vi "Save niVNA Sweep Data to csv.vi"(4 "Meas Type":string="QuickView_", 5 "Selected Exp Settings":T13={"P2_Sweep_Stop_V"=36.0, "P2_Sweep_Step_V"=1.0, "Experiment Name"="", "Resistance Threshold"=1.0, "P1_Fixed_Voltage"=36.0, "P2_Sweep_Start_V"=36.0}, 6 "Additional Data":T14, 7 "Filepath":path, 8 "Parametric Calculated Values":T5={"Voltage Calculated Values"={"P1_VPD_C"=0.0, "P2_VPD_C"=0.0, "P1_VPD_Rel_C"=0.0, "P2_VPD_Rel_C"=0.0}, "Resistance Calculated Values"={"Rc_free"=0.0, "Rc_first"=0.0, "Rc_vmax"=0.0, "Rc_last"=0.0, "Rc_end"=0.0, "VPD_R"=0.0, "VPD_Rel_R"=0.0}, "Capacitance Calculated Values"={"P1_CPD_free"=0.0, "P2_CPD_free"=0.0, "P1_CPD_vmax"=0.0, "P2_CPD_vmax"=0.0, "P1_CPD_first"=0.0, "P2_CPD_first"=0.0, "P1_CPD_last"=0.0, "P2_CPD_last"=0.0, "P1_CPD_end"=0.0, "P2_CPD_end"=0.0, "P1_CPD_max"=0.0, "P2_CPD_max "=0.0, "CPD_Free"=0.0, "CPD_First"=0.0, "CPD_max"=0.0, "CPD_Last"=0.0, "CPD_End"=0.0, "CPD_vmax"=0.0}, "Cap Calc Arrays"={"CPD_sum"=[], "P2_CPD@V"=[], "P1_CPD@V"=[], "Specific Voltages"=[32.0, 36.0]}, "Resistance Array Calc"={"RC@V"=[]}, "TN4 Calc"={"P1_TN4_ACT"=0.0, "P2_TN4_ACT "=0.0, "VPD_R_2"=0.0, "DVR"=0.0}, "Corrected_Capacitance Calculated Values"={"P1_CPD_free"=0.0, "P2_CPD_free"=0.0, "P1_CPD_vmax"=0.0, "P2_CPD_vmax"=0.0, "P1_CPD_first"=0.0, "P2_CPD_first"=0.0, "P1_CPD_last"=0.0, "P2_CPD_last"=0.0, "P1_CPD_end"=0.0, "P2_CPD_end"=0.0, "P1_CPD_max"=0.0, "P2_CPD_max "=0.0, "CPD_Free"=0.0, "CPD_First"=0.0, "CPD_max"=0.0, "CPD_Last"=0.0, "CPD_End"=0.0, "CPD_vmax"=0.0}}, 9 "ks5080A_Meaurements":T4, 10 "Date Cluster":T3, 11 "Test Information":T2={"Exp Name"="Cold Switching", "Lot"="0233A", "Wafer"="15", "Die Type"="L22", "Die X "="6", "Die Y"="8", "Exp"="1", "Die X_Y"="8"}) -> ()   [LabVIEW 2013]
uses:
  Controls/Date Control.ctl
  Controls/Individual User Inputs.ctl
  Controls/Test Information.ctl
  Controls/Parametric Calculated Values.ctl
  Controls/Voltage Calculated Values.ctl
  Controls/Resistance Individual Calculated Values.ctl
  Controls/Capacitance Individual Calculated Values.ctl
  Controls/Capacitance Array Calculated Values.ctl
  Controls/Resistance Array Calculated Values.ctl
  Controls/TN4 Calc.ctl
  Controls/Corrected_Capacitance Individual Calculated Values.ctl
  Controls/Additional Data.ctl
  Controls/ks5080A_Measurements.ctl
  <vilib>/Utility/file.llb/Write To Spreadsheet File (string).vi
panel:
  in  "Tab Control":T1(tab)
  # "Test Settings"
  # "Make the Stop and Step Negative \nfor negative sweep"
  # "Calculation Settings"
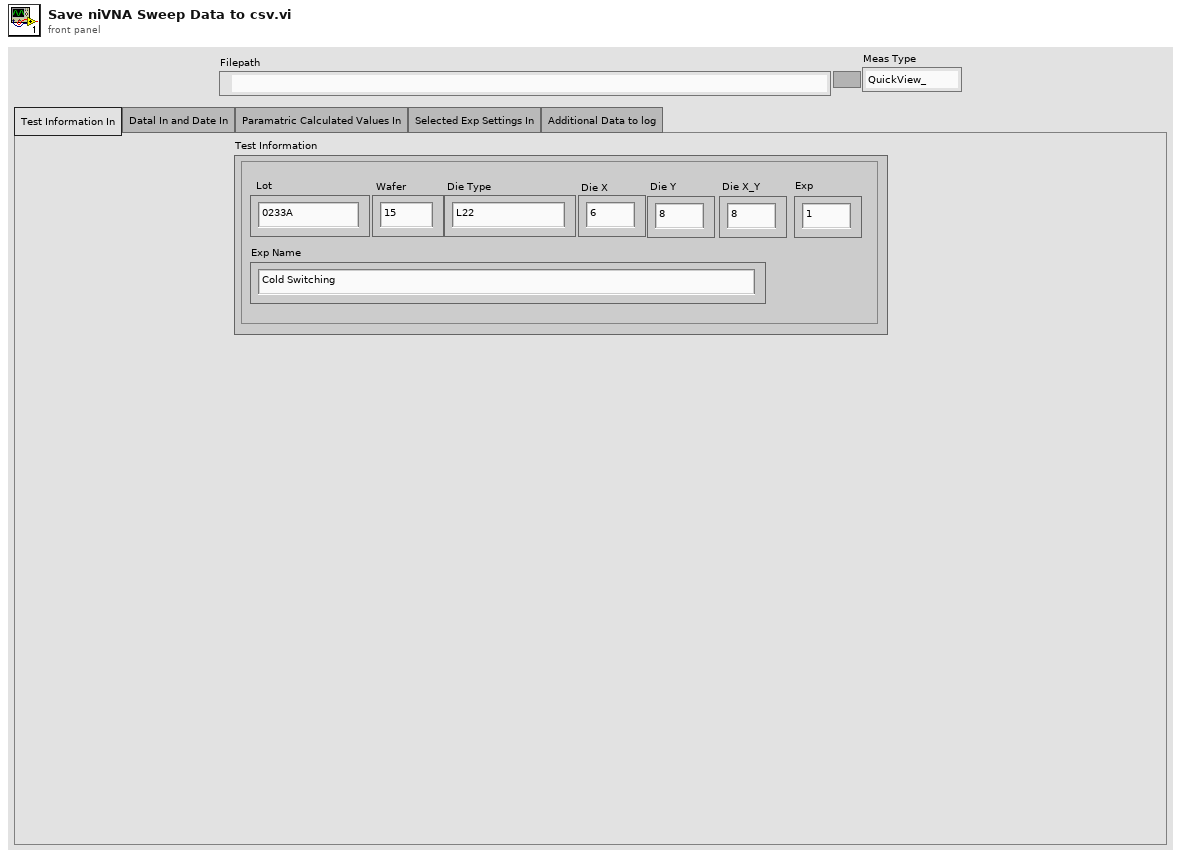
[diagram p1: front panel]
types:
  T1 = enum32{"Test Information In", "Datal In and Date In", "Paramatric Calculated Values In", "Selected Exp Settings In", "Additional Data to log"}
  T2 = typedef "Test Information.ctl" = cluster{"Exp Name":string, "Lot":string, "Wafer":string, "Die Type":string, "Die X ":string, "Die Y":string, "Exp":string, "Die X_Y":string}
  T3 = typedef "Date Control.ctl" = cluster{"Date":string, "Start Time":string, "Stop Time":string}
  T4 = typedef "ks5080A_Measurements.ctl" = cluster{"Bias_Sweep_Setting":dbl[], "Bias_voltage measurements":dbl[], "Bias_current measurements":dbl[], "P1_Capacitance":dbl[], "P2_Capacitance":dbl[], "DMM_Measurement_V":dbl[], "Contact_Source Current measurements":dbl[], "Contact_Sink Current measurements":dbl[], "Calculated_Resistance":dbl[], "P3_Capacitance":dbl[], "Port 1_S_parm":string[], "Port 2_S_parm":string[], "Port 3_S_parm":string[]}
  T5 = typedef "Parametric Calculated Values.ctl" = cluster{"Voltage Calculated Values":T6, "Resistance Calculated Values":T7, "Capacitance Calculated Values":T8, "Cap Calc Arrays":T9, "Resistance Array Calc":T10, "TN4 Calc":T11, "Corrected_Capacitance Calculated Values":T12}
  T6 = typedef "Voltage Calculated Values.ctl" = cluster{"P1_VPD_C":dbl, "P2_VPD_C":dbl, "P1_VPD_Rel_C":dbl, "P2_VPD_Rel_C":dbl}
  T7 = typedef "Resistance Individual Calculated Values.ctl" = cluster{"Rc_free":dbl, "Rc_first":dbl, "Rc_vmax":dbl, "Rc_last":dbl, "Rc_end":dbl, "VPD_R":dbl, "VPD_Rel_R":dbl}
  T8 = typedef "Capacitance Individual Calculated Values.ctl" = cluster{"P1_CPD_free":dbl, "P2_CPD_free":dbl, "P1_CPD_vmax":dbl, "P2_CPD_vmax":dbl, "P1_CPD_first":dbl, "P2_CPD_first":dbl, "P1_CPD_last":dbl, "P2_CPD_last":dbl, "P1_CPD_end":dbl, "P2_CPD_end":dbl, "P1_CPD_max":dbl, "P2_CPD_max ":dbl, "CPD_Free":dbl, "CPD_First":dbl, "CPD_max":dbl, "CPD_Last":dbl, "CPD_End":dbl, "CPD_vmax":dbl}
  T9 = typedef "Capacitance Array Calculated Values.ctl" = cluster{"CPD_sum":dbl[], "P2_CPD@V":dbl[], "P1_CPD@V":dbl[], "Specific Voltages":dbl[]}
  T10 = typedef "Resistance Array Calculated Values.ctl" = cluster{"RC@V":dbl[]}
  T11 = typedef "TN4 Calc.ctl" = cluster{"P1_TN4_ACT":dbl, "P2_TN4_ACT ":dbl, "VPD_R_2":dbl, "DVR":dbl}
  T12 = typedef "Corrected_Capacitance Individual Calculated Values.ctl" = cluster{"P1_CPD_free":dbl, "P2_CPD_free":dbl, "P1_CPD_vmax":dbl, "P2_CPD_vmax":dbl, "P1_CPD_first":dbl, "P2_CPD_first":dbl, "P1_CPD_last":dbl, "P2_CPD_last":dbl, "P1_CPD_end":dbl, "P2_CPD_end":dbl, "P1_CPD_max":dbl, "P2_CPD_max ":dbl, "CPD_Free":dbl, "CPD_First":dbl, "CPD_max":dbl, "CPD_Last":dbl, "CPD_End":dbl, "CPD_vmax":dbl}
  T13 = typedef "Individual User Inputs.ctl" = cluster{"P2_Sweep_Stop_V":dbl, "P2_Sweep_Step_V":dbl, "Experiment Name":string, "Resistance Threshold":dbl, "P1_Fixed_Voltage":dbl, "P2_Sweep_Start_V":dbl}
  T14 = typedef "Additional Data.ctl" = cluster{"P2_Capacitance_PostTest":dbl[], "P1_Capacitance _PostTest":dbl[], "P1_Capacitance_PreTest":dbl[], "P2_Capacitance_PreTest":dbl[]}
  T15 = enum16{"open", "replace", "create", "open or create", "replace or create", "replace or create with confirmation"}
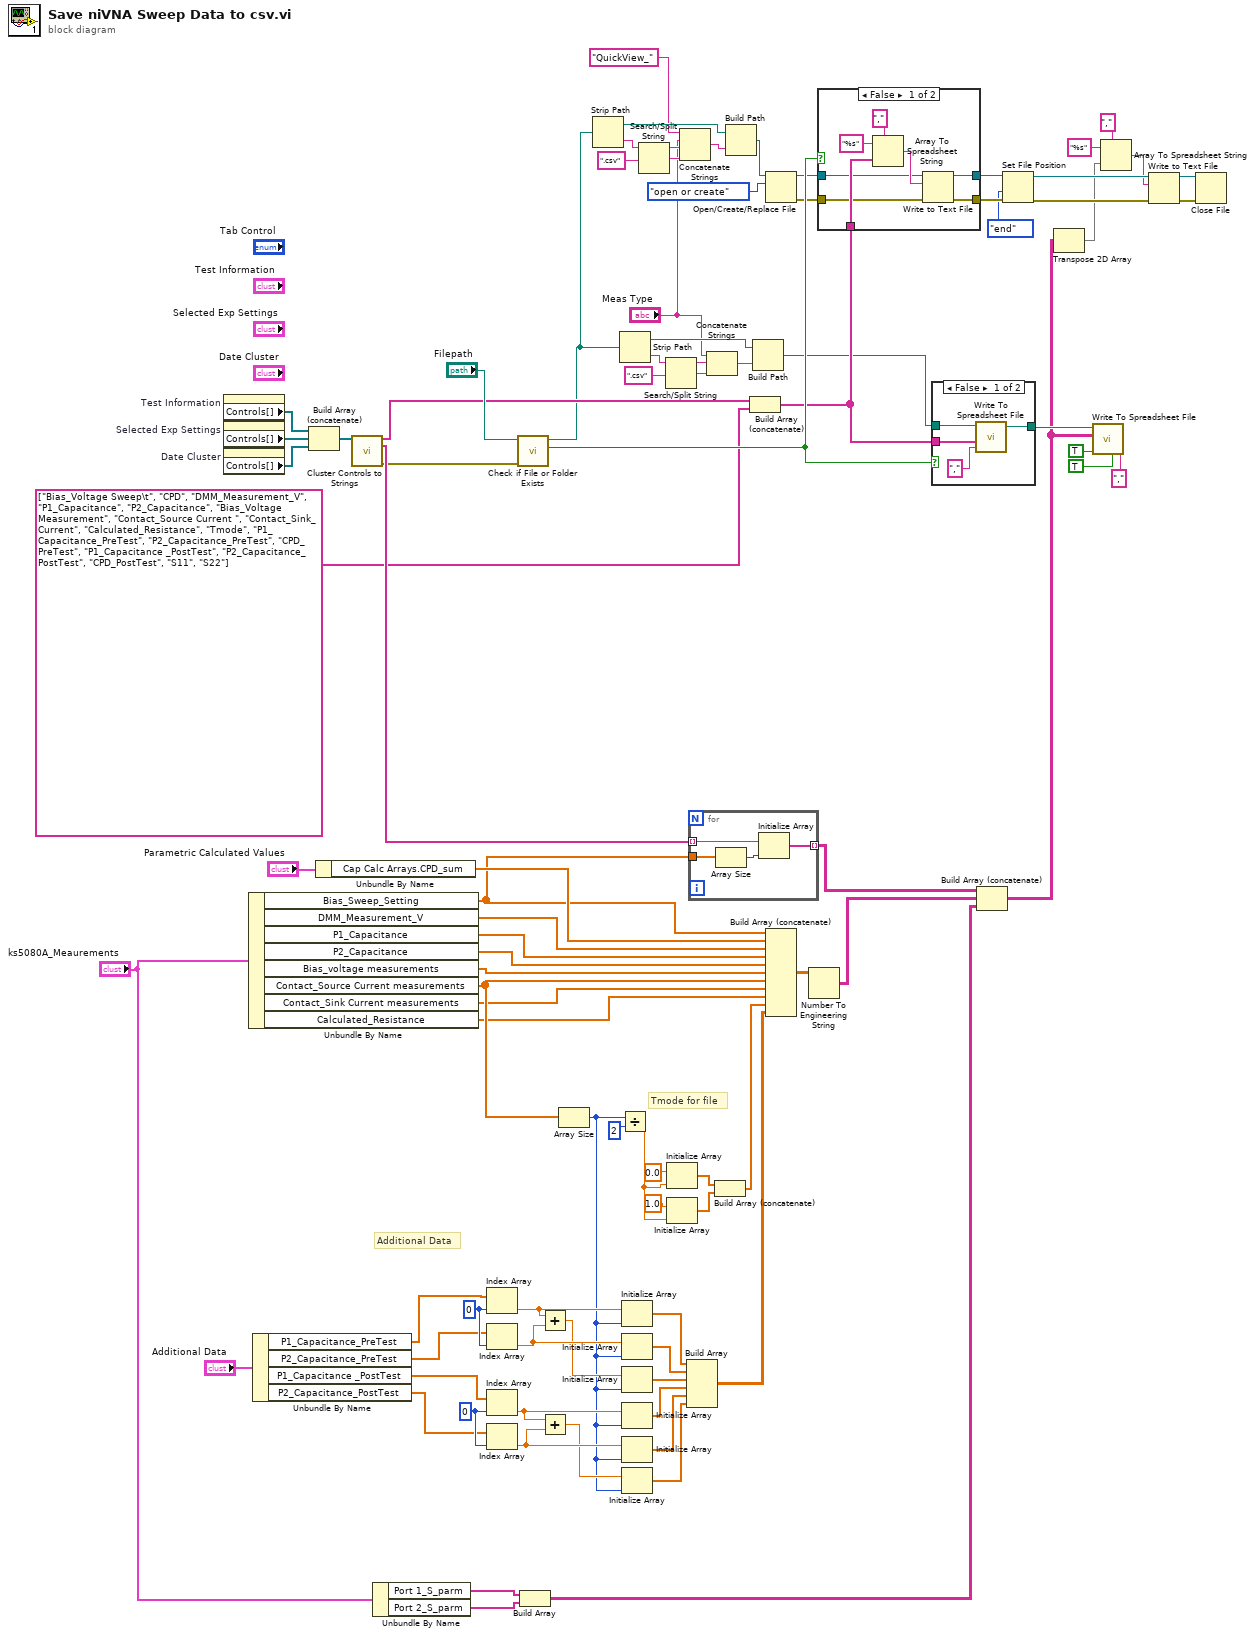
[diagram p0: block diagram]
diagram:
  w43 = 0 ("index")
  w44 = 0 ("index")
  # "Additional Data"
  # "Tmode for file"
  n1 = property on="Test Information" class="Clust (strict)"() -> ("Controls[]"=w92:refnum<vi>[])  [unwired: 2 in, 2 out]
  n2 = property on="Selected Exp Settings" class="Clust (strict)"() -> ("Controls[]"=w91:refnum<vi>[])  [unwired: 2 in, 2 out]
  n3 = property on="Date Cluster" class="Clust (strict)"() -> ("Controls[]"=w89:refnum<vi>[])  [unwired: 2 in, 2 out]
  n4 = Unbundle By Name("ks5080A_Meaurements") -> ("Bias_Sweep_Setting"=w15:dbl[], "DMM_Measurement_V"=w14:dbl[], "P1_Capacitance"=w13:dbl[], "P2_Capacitance"=w12:dbl[], "Bias_voltage measurements"=w11:dbl[], "Contact_Source Current measurements"=w10:dbl[], "Contact_Sink Current measurements"=w9:dbl[], "Calculated_Resistance"=w8:dbl[])
  n5 = Unbundle By Name("Additional Data") -> ("P1_Capacitance_PreTest"=w27:dbl[], "P2_Capacitance_PreTest"=w26:dbl[], "P1_Capacitance _PostTest"=w25:dbl[], "P2_Capacitance_PostTest"=w24:dbl[])
  n6 = Build Array (concatenate)(w92, w91, w89) -> (w90:refnum<vi>[])
  n7 = Unbundle By Name("Parametric Calculated Values") -> ("Cap Calc Arrays.CPD_sum"=w70:dbl[])
  n8 = call "Cluster Controls to Strings.vi"("Controls[]"=w90) -> ("Control Labels"=w73:string[], "Control Values"=w88:string[], "Error Out"=w72:errorcluster)  [unwired: 12 in]
  n9 = Unbundle By Name("ks5080A_Meaurements") -> ("Port 1_S_parm"=w6:string[], "Port 2_S_parm"=w5:string[])
  n10 = Index Array(array=w27, index=w44) -> (element=w42:dbl)
  n11 = Index Array(array=w26, index=w44) -> (element=w41:dbl)
  n12 = Index Array(array=w25, index=w43) -> (element=w39:dbl)
  n13 = Index Array(array=w24, index=w43) -> (element=w38:dbl)
  n14 = call <vilib>:"Check if File or Folder Exists.vi"("error in (no error)"=w72, "path"="Filepath") -> ("file or folder exists?"=w61:bool, "dup path"=w17:path)  [unwired: 7 in, 1 out]
  n15 = Build Array(w6, w5) -> (w4:string[][])
  n16 = Add(x=w42, y=w41) -> (x+y=w40:dbl)
  n17 = Add(x=w39, y=w38) -> (x+y=w37:dbl)
  n18 = Array Size(array=w10) -> (size(s)=w36:i32)
  n19 = Strip Path(path=w17) -> (stripped path=w65:path, name=w68:string)
  n20 = Strip Path(path=w17) -> (stripped path=w20:path, name=w23:string)
  n21 = Divide(x=w36, y=2) -> (x/y=w86:dbl)
  n22 = Initialize Array(w42, w36) -> (w35:dbl[])
  n23 = Initialize Array(w41, w36) -> (w34:dbl[])
  n24 = Initialize Array(w40, w36) -> (w33:dbl[])
  n25 = Initialize Array(w39, w36) -> (w32:dbl[])
  n26 = Initialize Array(w38, w36) -> (w31:dbl[])
  n27 = Initialize Array(w37, w36) -> (w30:dbl[])
  n28 = Search/Split String(string=w68, search string/char (-)=".csv" ("search string")) -> (substring before match=w63:string, match + rest of string=w66:string)  [unwired: 1 in, 1 out]
  n29 = Search/Split String(string=w23, search string/char (-)=".csv" ("search string")) -> (substring before match=w18:string, match + rest of string=w21:string)  [unwired: 1 in, 1 out]
  n30 = Initialize Array(0.0, w86) -> (w87:dbl[])
  n31 = Initialize Array(1.0, w86) -> (w82:dbl[])
  n32 = Concatenate Strings("QuickView_" ("search string"), "Meas Type", w63, w66) -> (w64:string)
  n33 = Build Array(w35, w34, w33, w32, w31, w30) -> (w29:dbl[][])
  n34 = for {
    tunnel: w15 -> [w96]
    tunnel: w88 -> [w95] mode=indexing
    tunnel: [w93] -> w77 mode=indexing
    n35 = Array Size(array=w96) -> (size(s)=w94:i32)
    n36 = Initialize Array(w95, w94) -> (w93:string[])
  }
  n37 = Concatenate Strings("Meas Type", w18, w21) -> (w19:string)
  n38 = Build Array (concatenate)(w87, w82) -> (w45:dbl[])
  n39 = Build Path(base path=w65, name or relative path=w64) -> (appended path=w62:path)
  n40 = Build Array (concatenate)(w73, string[] ["Bias_Voltage Sweep\t", "CPD", "DMM_Measurement_V", "P1_Capacitance", "P2_Capacitance", "Bias_Voltage Measurement", "Contact_Source Current ", "Contact_Sink_Current", "Calculated_Resistance", "Tmode", "P1_Capacitance_PreTest", "P2_Capacitance_PreTest", "CPD_PreTest", "P1_Capacitance _PostTest", "P2_Capacitance_PostTest", "CPD_PostTest", "S11", "S22"]) -> (w60:string[])
  n41 = Build Path(base path=w20, name or relative path=w19) -> (appended path=w16:path)
  n42 = Open/Create/Replace File(file path (use dialog)=w62, operation (0:open)=T15."open or create") -> (refnum out=w59:refnum<file>, error out=w58:errorcluster)  [unwired: 4 in, 1 out]
  n43 = Build Array (concatenate)(w15, w70, w14, w13, w12, w11, w10, w9, w8, w45, w29) -> (w75:dbl[][])
  n44 = Number To Engineering String(4:w75) -> (0:w76:string[][])  [unwired: 3 in]
  n45 = case shown="False" w61 {
    tunnel: w60 -> [w102 _]
    tunnel: w59 -> [w100 w106]
    tunnel: w58 -> [w99 w105]
    tunnel: [w98 w105] -> w56
    tunnel: [w97 w106] -> w57
    frame False {
      n46 = Array To Spreadsheet String(delimiter (Tab)="," ("delimiter (\\t)"), array=w102, 3:"%s" ("format string")) -> (spreadsheet string=w101:string)
      n47 = Write to Text File(file (use dialog)=w100, text=w101, error in=w99) -> (refnum out=w97:refnum<file>, error out=w98:errorcluster)  [unwired: 1 in, 1 out]
    }
    frame True {
    }
  }
  n48 = case shown="False" w61 {
    tunnel: w16 -> [w110 w111]
    tunnel: w60 -> [w109 _]
    tunnel: [w107 w111] -> w81
    frame False {
      n49 = call-poly <vilib>:"Write To Spreadsheet File.vi"("delimiter (\\t)"="," ("delimiter (\\t)"), "1D data"=w109, "file path (dialog if empty)"=w110) -> ("new file path (Not A Path if cancelled)"=w107:path)  [unwired: 5 in]
    }
    frame True {
    }
  }
  n50 = Build Array (concatenate)(w77, w76, w4) -> (w47:string[][])
  n51 = Set File Position(refnum=w57, from (0:start)=enum16{"start", "end", "current"}."end", error in=w56) -> (refnum out=w51:refnum<file>, error out=w52:errorcluster)  [unwired: 1 in]
  n52 = Transpose 2D Array(2D array=w47) -> (transposed array=w46:string[][])
  n53 = call-poly <vilib>:"Write To Spreadsheet File.vi"("delimiter (\\t)"="," ("delimiter (\\t)"), "transpose? (no:F)"=TRUE, "append to file? (new file:F)"=TRUE, "2D data"=w47, "file path (dialog if empty)"=w81) -> ()  [unwired: 3 in, 1 out]
  n54 = Array To Spreadsheet String(delimiter (Tab)="," ("delimiter (\\t)"), array=w46, 3:"%s" ("format string")) -> (spreadsheet string=w50:string)
  n55 = Write to Text File(file (use dialog)=w51, text=w50, error in=w52) -> (refnum out=w48:refnum<file>, error out=w49:errorcluster)  [unwired: 1 in, 1 out]
  n56 = Close File(refnum=w48, error in=w49) -> ()  [unwired: 2 out]
